vi "Release Logger.vi"(8 "error in (no error)":errorcluster, 11 "Producer":refnum<class "Log Producer.lvclass">) -> (0 "error out":errorcluster, 3 "Default Producer":refnum<class "Log Producer.lvclass">)   [LabVIEW 2020, in "AIM ARINC 429 Engine.lvlib" / "Implementation.lvlib" / "Word Logging.lvlib"]
uses:
  Word Logging.lvlib
  Log Producer/Log Producer.lvclass
  C:/Program Files (x86)/National Instruments/LabVIEW 2020/vi.lib/NI/VeriStand Custom Device Messaging/Producer/Abstract Producer/Abstract Producer.lvclass
  <vilib>/NI/VeriStand Custom Device Messaging/Message/Shutdown Message/Shutdown Message.lvclass
  C:/Program Files (x86)/National Instruments/LabVIEW 2020/vi.lib/NI/VeriStand Custom Device Messaging/Message/Abstract Message/Abstract Message.lvclass
  <vilib>/NI/VeriStand Custom Device Messaging/Producer/Abstract Producer/Abstract Producer.lvclass
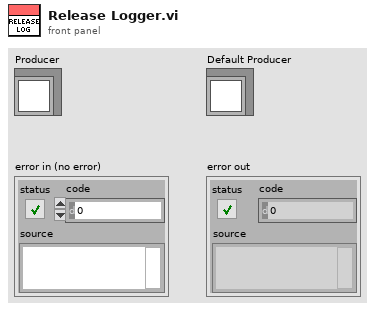
[diagram p1: front panel]
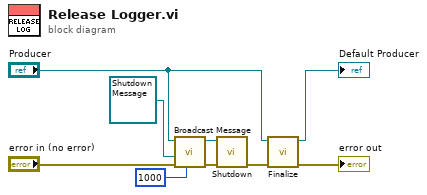
[diagram p0: block diagram]
diagram:
  n1 = call-dynamic "Broadcast Message.vi"("timeout in ms (-1)"=1000, "error in (no error)"="error in (no error)", "Message in"=refnum<class "Shutdown Message.lvclass"> refnum ("Messaging.lvlib:Shutdown Message.lvclass"), "Abstract Producer in"="Producer") -> ("error out"=w7:errorcluster, "Abstract Producer out"=w5:refnum<class "Log Producer.lvclass">)  [unwired: 4 in, 2 out]
  n2 = call <vilib>:"Shutdown.vi"("error in (no error)"=w7, "Abstract Producer in"=w5) -> ("error out"=w6:errorcluster)  [unwired: 8 in, 1 out]
  n3 = call "Finalize.vi"("error in (no error)"=w6, "Log Producer"="Producer") -> ("error out"=→"error out":errorcluster, "Default Producer"=→"Default Producer":refnum<class "Log Producer.lvclass">)  [unwired: 7 in, 1 out]
